vi "Inventory.vi"(8 "error in (no error)":errorcluster, 11 "Productos in":refnum<class "Productos.lvclass">) -> (0 "error out":errorcluster, 2 "Productos 2":T1, 3 "Productos out":refnum<class "Productos.lvclass">)   [LabVIEW 2020, in "Productos.lvlib" / "Productos.lvclass"]
uses:
  Productos.lvclass
panel:
  in  "Productos":T1
  in  "Cancel Button":bool
  in  "OK Button":bool
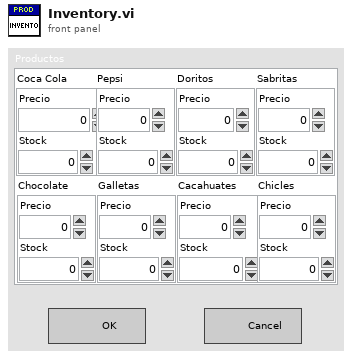
[diagram p1: front panel]
types:
  T1 = cluster{"Coca Cola":cluster{"Precio":dbl, "Stock":dbl}, "Pepsi":cluster{"Precio":dbl, "Stock":dbl}, "Doritos":cluster{"Precio":dbl, "Stock":dbl}, "Sabritas":cluster{"Precio":dbl, "Stock":dbl}, "Chocolate":cluster{"Precio":dbl, "Stock":dbl}, "Galletas":cluster{"Precio":dbl, "Stock":dbl}, "Cacahuates":cluster{"Precio":dbl, "Stock":dbl}, "Chicles":cluster{"Precio":dbl, "Stock":dbl}}
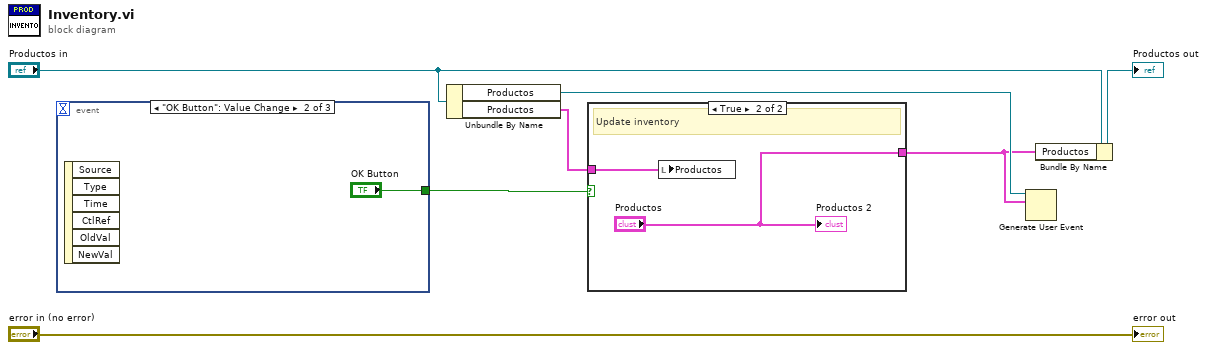
[diagram p0: block diagram]
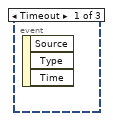
[diagram p3: hidden frame]
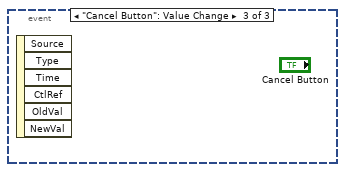
[diagram p4: hidden frame]
diagram:
  n1 = event shown="[1] \"OK Button\": Value Change" {
    selector: _ -> [_ _ _]
    dyn-events: _ -> [_ _ _]
    timeout: _ -> [_ _ _]
    tunnel: [_ "OK Button" _] -> w6
    event Timeout {
      n2 = event-data() -> ()  [unwired: 1 in, 3 out]
    }
    event "OK Button": Value Change {
      n3 = event-data() -> ()  [unwired: 1 in, 6 out]
    }
    event "Cancel Button": Value Change {
      n4 = event-data() -> ()  [unwired: 1 in, 6 out]
    }
  }
  n5 = Unbundle By Name("Productos in") -> ("Productos"=w3:refnum<user-event>, "Productos"=w1:T1)
  n6 = case shown="True" w6 {
    tunnel: [_ "Productos"] -> w2
    tunnel: w1 -> [_ w9]
    frame False {
    }
    frame True {
      # "Update inventory"
      n7 = local write "Productos"(w9) -> ()
      "Productos 2" <- "Productos"
    }
  }
  n8 = Generate User Event(user event=w3, event data cluster=w2) -> ()  [unwired: 2 in, 2 out]
  n9 = Bundle By Name(cluster="Productos in", "Productos"=w2) -> (→"Productos out":refnum<class "Productos.lvclass">)
  "error out" <- "error in (no error)"
